vi "linear interp -- residue.vi"(7 "what":enum16{"linear", "quadratic", "nothing"}(ring), 10 "what points in":dbl[](array[numeric])=[-1.4233131928950045, -1.44696698189356, -1.4387793191620561, -1.4336803765711887, -1.4766437914412072, -1.4238891039751602, -1.4266641580299324, -1.4249276723821875, -1.4343882731939412, -1.4156687737284692, -1.4512421695222957, -1.429807437000274, -1.4155556909308238, -1.4387793191620561, -1.4256214336829176, -1.4378261347313517, -1.472241245575028, -1.476513665752772, -1.4669909756005146, -1.430275048869841, -1.4314462860465573, -1.4375881651462725, -1.4885177094699984, -1.3721223035160284, -1.4390179425097644, -1.430626088480954, -1.4084901891013457, -1.4885177094699984, -1.430275048869841, -1.4816176825506562, -1.4117282912536708, -1.420102128492896, -1.414200989082999, -1.4412914275628341, -1.4275931305379441, -1.4362816581303222, -1.4294570582141024, -1.449038245797824, -1.4286406053421603, -1.431211785780653, -1.4307431647673898, -1.430626088480954, -1.4310945831131212, -1.4301580986922384, -1.4330913428691965, -1.5284149439108103, -1.450996736070212, -1.449404790606672, -1.4596705233051261, -1.4422522564545317, -1.4500163869363112, -1.4513649382812484, -1.4485500001231248, -1.4439388390864674, -1.4579218517603743, -1.4631891321044586, -1.465593098958123, -1.4559319537457243, -1.4673729968671088, -1.447210147903218, -1.447696888757646, -1.4348608461262105, -1.447696888757646, -1.4373503258840832, -1.438898614446944, -1.4737899942543355, -1.4484280244217462, -1.4242350175592806, -1.4386600566370986, -1.5039010059634286, -1.4487940543480937, -1.4347426546757862, -1.4293403280744659, -1.4346244953819263, -1.4560560556130935, -1.486382924308125, -1.4525945384285102, -1.5065419471008115, -1.4360445331001872, -1.4326206904450212, -1.4059390968255816, -1.4248121531683389, -1.4270122898977948, -1.4435768767247146, -1.447696888757646, -1.4271283958955197, -1.4268962149320088, -1.4462382997059955, -1.4219341142599085, -1.425968730368281, -1.438540826854084, -1.423773860646395, -1.4007721353222036, -1.4364002692144688, -1.4378261347313517, -1.4333268604898834, -1.4255057298106724, -1.4776862029393325, -1.4273607010531868, -1.4207882178645008, -1.4189610493238327, -1.42969061266012, -1.4112802184959434, -1.4282911662873123, -1.4605475065465392, -1.4270122898977948, -1.394479474658531, -1.4281747490551708, -1.4212462136695654, -1.4236586478902071, -1.407823240700133, -1.4039529905505608, -1.4082677591441644, -1.4256214336829176, -1.41016205494854, -1.4115041970887898, -1.413187728652624, -1.411840381712908, -1.404944908336696, -1.4094925360874166, -1.4263163050022019, -1.4189610493238327, -1.4191890254350537, -1.4124012683747549, -1.4031830621804093, -1.4027437151708582, -1.399462703731531, -1.4038429171798275, -1.4124012683747549, -1.4015377976218495, -1.3966390737476193, -1.4086014468147512, -1.3976144079908948, -1.398265849835895, -1.4081565868712154, -1.3873220797794983, -1.396206293959037, -1.4042833781525756, -1.3759242669503173, -1.3791355228308788, -1.384365529218584, -1.4086014468147512, -1.3885953603844066, -1.402633947829972, -1.3902988957166005, -1.3972890531384425, -1.400007820511902, -1.3731465834292742, -1.376440608090563, -1.4293403280744659, -1.3726341415032672, -1.3798639431222424, -1.3880643730558775, -1.3630108962837708, -1.3713046153819766, -1.392009139548825, -1.3360165434877334, -1.3750993958915096, -1.3514448424333292, -1.3759242669503173, -1.372224622866697, -1.3371477648312038, -1.3381873125587387, -1.3768541234580602, -1.3643152355487773, -1.3590219407376678, -1.3521282327897675, -1.3731465834292742, -1.3689623015592596, -1.3502758121664775, -1.3365817858433202, -1.3120253780614444, -1.3605135088274138, -1.3602147851091797, -1.3516399871150684, -1.3737623129490995, -1.35261702798138, -1.3653212459173176, -1.351835219521999, -1.3320803127786385, -1.372736581527779, -1.410608974959067, -1.3461124400250224, -1.4067139310755428, -1.308830063964396, -1.3486250541829568, -1.3950183684885684, -1.349304018335389, -1.3283644014938703, -1.3056580877318187, -1.3363932899714797, -1.3342314473766201, -1.3269790909671038, -1.3485281458969576, -1.3613111114058765, -1.3408447171553701, -1.330962197210844, -1.324863493628006, -1.3103360330802296, -1.3067128410903444, -1.3183969993651314, -1.3216637513638199, -1.32947584031392, -1.3245883043811366], 11 "temperature points in":dbl[](array[numeric])=[55.393, 55.473, 55.549, 55.623, 55.697, 55.77, 55.847, 55.926, 56.007, 56.087, 56.169, 56.251, 56.332, 56.409, 56.489, 56.565, 56.645, 56.724, 56.8, 56.877, 56.955, 57.034, 57.114, 57.191, 57.269, 57.348, 57.425, 57.505, 57.583, 57.656, 57.736, 57.815, 57.896, 57.974, 58.055, 58.137, 58.217, 58.295, 58.373, 58.45, 58.526, 58.605, 58.679, 58.759, 58.836, 58.913, 58.989, 59.071, 59.148, 59.226, 59.302, 59.381, 59.459, 59.539, 59.616, 59.694, 59.77, 59.846, 59.925, 59.998, 60.076, 60.154, 60.23, 60.308, 60.384, 60.462, 60.54, 60.618, 60.693, 60.77, 60.849, 60.928, 61.004, 61.082, 61.16, 61.239, 61.315, 61.391, 61.468, 61.544, 61.626, 61.703, 61.781, 61.86, 61.93, 62.009, 62.083, 62.162, 62.238, 62.312, 62.389, 62.466, 62.541, 62.618, 62.697, 62.774, 62.854, 63.013, 63.088, 63.165, 63.241, 63.317, 63.394, 63.472, 63.549, 63.628, 63.705, 63.782, 63.861, 63.937, 64.014, 64.089, 64.162, 64.239, 64.316, 64.393, 64.47, 64.547, 64.62, 64.696, 64.817, 64.892, 64.971, 65.046, 65.123, 65.2, 65.275, 65.35, 65.429, 65.507, 65.582, 65.655, 65.733, 65.81, 65.887, 65.965, 66.042, 66.193, 66.27, 66.345, 66.423, 66.5, 66.574, 66.651, 66.728, 66.802, 66.881, 66.956, 67.032, 67.108, 67.187, 67.258, 67.335, 67.411, 67.487, 67.563, 67.639, 67.717, 67.792, 67.869, 67.941, 68.018, 68.097, 68.174, 68.251, 68.349, 68.484, 68.558, 68.632, 68.708, 68.787, 68.864, 69.014, 69.092, 69.169, 69.246, 69.323, 69.397, 69.472, 69.546, 69.621, 69.696, 69.771, 69.845, 69.924, 69.997, 70.071, 70.149, 70.225, 70.301, 70.381, 70.457, 70.533, 70.609, 70.682, 70.76, 70.84, 70.915, 70.993, 71.145, 71.222, 71.3, 71.374, 71.452]) -> (0 "resudue points out":dbl[](array[numeric])=[-1.4233131928950045, -1.44696698189356, -1.4387793191620561, -1.4336803765711887, -1.4766437914412072, -1.4238891039751602, -1.4266641580299324, -1.4249276723821875, -1.4343882731939412, -1.4156687737284692, -1.4512421695222957, -1.429807437000274, -1.4155556909308238, -1.4387793191620561, -1.4256214336829176, -1.4378261347313517, -1.472241245575028, -1.476513665752772, -1.4669909756005146, -1.430275048869841, -1.4314462860465573, -1.4375881651462725, -1.4885177094699984, -1.3721223035160284, -1.4390179425097644, -1.430626088480954, -1.4084901891013457, -1.4885177094699984, -1.430275048869841, -1.4816176825506562, -1.4117282912536708, -1.420102128492896, -1.414200989082999, -1.4412914275628341, -1.4275931305379441, -1.4362816581303222, -1.4294570582141024, -1.449038245797824, -1.4286406053421603, -1.431211785780653, -1.4307431647673898, -1.430626088480954, -1.4310945831131212, -1.4301580986922384, -1.4330913428691965, -1.5284149439108103, -1.450996736070212, -1.449404790606672, -1.4596705233051261, -1.4422522564545317, -1.4500163869363112, -1.4513649382812484, -1.4485500001231248, -1.4439388390864674, -1.4579218517603743, -1.4631891321044586, -1.465593098958123, -1.4559319537457243, -1.4673729968671088, -1.447210147903218, -1.447696888757646, -1.4348608461262105, -1.447696888757646, -1.4373503258840832, -1.438898614446944, -1.4737899942543355, -1.4484280244217462, -1.4242350175592806, -1.4386600566370986, -1.5039010059634286, -1.4487940543480937, -1.4347426546757862, -1.4293403280744659, -1.4346244953819263, -1.4560560556130935, -1.486382924308125, -1.4525945384285102, -1.5065419471008115, -1.4360445331001872, -1.4326206904450212, -1.4059390968255816, -1.4248121531683389, -1.4270122898977948, -1.4435768767247146, -1.447696888757646, -1.4271283958955197, -1.4268962149320088, -1.4462382997059955, -1.4219341142599085, -1.425968730368281, -1.438540826854084, -1.423773860646395, -1.4007721353222036, -1.4364002692144688, -1.4378261347313517, -1.4333268604898834, -1.4255057298106724, -1.4776862029393325, -1.4273607010531868, -1.4207882178645008, -1.4189610493238327, -1.42969061266012, -1.4112802184959434, -1.4282911662873123, -1.4605475065465392, -1.4270122898977948, -1.394479474658531, -1.4281747490551708, -1.4212462136695654, -1.4236586478902071, -1.407823240700133, -1.4039529905505608, -1.4082677591441644, -1.4256214336829176, -1.41016205494854, -1.4115041970887898, -1.413187728652624, -1.411840381712908, -1.404944908336696, -1.4094925360874166, -1.4263163050022019, -1.4189610493238327, -1.4191890254350537, -1.4124012683747549, -1.4031830621804093, -1.4027437151708582, -1.399462703731531, -1.4038429171798275, -1.4124012683747549, -1.4015377976218495, -1.3966390737476193, -1.4086014468147512, -1.3976144079908948, -1.398265849835895, -1.4081565868712154, -1.3873220797794983, -1.396206293959037, -1.4042833781525756, -1.3759242669503173, -1.3791355228308788, -1.384365529218584, -1.4086014468147512, -1.3885953603844066, -1.402633947829972, -1.3902988957166005, -1.3972890531384425, -1.400007820511902, -1.3731465834292742, -1.376440608090563, -1.4293403280744659, -1.3726341415032672, -1.3798639431222424, -1.3880643730558775, -1.3630108962837708, -1.3713046153819766, -1.392009139548825, -1.3360165434877334, -1.3750993958915096, -1.3514448424333292, -1.3759242669503173, -1.372224622866697, -1.3371477648312038, -1.3381873125587387, -1.3768541234580602, -1.3643152355487773, -1.3590219407376678, -1.3521282327897675, -1.3731465834292742, -1.3689623015592596, -1.3502758121664775, -1.3365817858433202, -1.3120253780614444, -1.3605135088274138, -1.3602147851091797, -1.3516399871150684, -1.3737623129490995, -1.35261702798138, -1.3653212459173176, -1.351835219521999, -1.3320803127786385, -1.372736581527779, -1.410608974959067, -1.3461124400250224, -1.4067139310755428, -1.308830063964396, -1.3486250541829568, -1.3950183684885684, -1.349304018335389, -1.3283644014938703, -1.3056580877318187, -1.3363932899714797, -1.3342314473766201, -1.3269790909671038, -1.3485281458969576, -1.3613111114058765, -1.3408447171553701, -1.330962197210844, -1.324863493628006, -1.3103360330802296, -1.3067128410903444, -1.3183969993651314, -1.3216637513638199, -1.32947584031392, -1.3245883043811366], 2 "what points out":dbl[](array[numeric])=[-1.4233131928950045, -1.44696698189356, -1.4387793191620561, -1.4336803765711887, -1.4766437914412072, -1.4238891039751602, -1.4266641580299324, -1.4249276723821875, -1.4343882731939412, -1.4156687737284692, -1.4512421695222957, -1.429807437000274, -1.4155556909308238, -1.4387793191620561, -1.4256214336829176, -1.4378261347313517, -1.472241245575028, -1.476513665752772, -1.4669909756005146, -1.430275048869841, -1.4314462860465573, -1.4375881651462725, -1.4885177094699984, -1.3721223035160284, -1.4390179425097644, -1.430626088480954, -1.4084901891013457, -1.4885177094699984, -1.430275048869841, -1.4816176825506562, -1.4117282912536708, -1.420102128492896, -1.414200989082999, -1.4412914275628341, -1.4275931305379441, -1.4362816581303222, -1.4294570582141024, -1.449038245797824, -1.4286406053421603, -1.431211785780653, -1.4307431647673898, -1.430626088480954, -1.4310945831131212, -1.4301580986922384, -1.4330913428691965, -1.5284149439108103, -1.450996736070212, -1.449404790606672, -1.4596705233051261, -1.4422522564545317, -1.4500163869363112, -1.4513649382812484, -1.4485500001231248, -1.4439388390864674, -1.4579218517603743, -1.4631891321044586, -1.465593098958123, -1.4559319537457243, -1.4673729968671088, -1.447210147903218, -1.447696888757646, -1.4348608461262105, -1.447696888757646, -1.4373503258840832, -1.438898614446944, -1.4737899942543355, -1.4484280244217462, -1.4242350175592806, -1.4386600566370986, -1.5039010059634286, -1.4487940543480937, -1.4347426546757862, -1.4293403280744659, -1.4346244953819263, -1.4560560556130935, -1.486382924308125, -1.4525945384285102, -1.5065419471008115, -1.4360445331001872, -1.4326206904450212, -1.4059390968255816, -1.4248121531683389, -1.4270122898977948, -1.4435768767247146, -1.447696888757646, -1.4271283958955197, -1.4268962149320088, -1.4462382997059955, -1.4219341142599085, -1.425968730368281, -1.438540826854084, -1.423773860646395, -1.4007721353222036, -1.4364002692144688, -1.4378261347313517, -1.4333268604898834, -1.4255057298106724, -1.4776862029393325, -1.4273607010531868, -1.4207882178645008, -1.4189610493238327, -1.42969061266012, -1.4112802184959434, -1.4282911662873123, -1.4605475065465392, -1.4270122898977948, -1.394479474658531, -1.4281747490551708, -1.4212462136695654, -1.4236586478902071, -1.407823240700133, -1.4039529905505608, -1.4082677591441644, -1.4256214336829176, -1.41016205494854, -1.4115041970887898, -1.413187728652624, -1.411840381712908, -1.404944908336696, -1.4094925360874166, -1.4263163050022019, -1.4189610493238327, -1.4191890254350537, -1.4124012683747549, -1.4031830621804093, -1.4027437151708582, -1.399462703731531, -1.4038429171798275, -1.4124012683747549, -1.4015377976218495, -1.3966390737476193, -1.4086014468147512, -1.3976144079908948, -1.398265849835895, -1.4081565868712154, -1.3873220797794983, -1.396206293959037, -1.4042833781525756, -1.3759242669503173, -1.3791355228308788, -1.384365529218584, -1.4086014468147512, -1.3885953603844066, -1.402633947829972, -1.3902988957166005, -1.3972890531384425, -1.400007820511902, -1.3731465834292742, -1.376440608090563, -1.4293403280744659, -1.3726341415032672, -1.3798639431222424, -1.3880643730558775, -1.3630108962837708, -1.3713046153819766, -1.392009139548825, -1.3360165434877334, -1.3750993958915096, -1.3514448424333292, -1.3759242669503173, -1.372224622866697, -1.3371477648312038, -1.3381873125587387, -1.3768541234580602, -1.3643152355487773, -1.3590219407376678, -1.3521282327897675, -1.3731465834292742, -1.3689623015592596, -1.3502758121664775, -1.3365817858433202, -1.3120253780614444, -1.3605135088274138, -1.3602147851091797, -1.3516399871150684, -1.3737623129490995, -1.35261702798138, -1.3653212459173176, -1.351835219521999, -1.3320803127786385, -1.372736581527779, -1.410608974959067, -1.3461124400250224, -1.4067139310755428, -1.308830063964396, -1.3486250541829568, -1.3950183684885684, -1.349304018335389, -1.3283644014938703, -1.3056580877318187, -1.3363932899714797, -1.3342314473766201, -1.3269790909671038, -1.3485281458969576, -1.3613111114058765, -1.3408447171553701, -1.330962197210844, -1.324863493628006, -1.3103360330802296, -1.3067128410903444, -1.3183969993651314, -1.3216637513638199, -1.32947584031392, -1.3245883043811366], 3 "temperature points OUT":dbl[](array[numeric])=[55.393, 55.473, 55.549, 55.623, 55.697, 55.77, 55.847, 55.926, 56.007, 56.087, 56.169, 56.251, 56.332, 56.409, 56.489, 56.565, 56.645, 56.724, 56.8, 56.877, 56.955, 57.034, 57.114, 57.191, 57.269, 57.348, 57.425, 57.505, 57.583, 57.656, 57.736, 57.815, 57.896, 57.974, 58.055, 58.137, 58.217, 58.295, 58.373, 58.45, 58.526, 58.605, 58.679, 58.759, 58.836, 58.913, 58.989, 59.071, 59.148, 59.226, 59.302, 59.381, 59.459, 59.539, 59.616, 59.694, 59.77, 59.846, 59.925, 59.998, 60.076, 60.154, 60.23, 60.308, 60.384, 60.462, 60.54, 60.618, 60.693, 60.77, 60.849, 60.928, 61.004, 61.082, 61.16, 61.239, 61.315, 61.391, 61.468, 61.544, 61.626, 61.703, 61.781, 61.86, 61.93, 62.009, 62.083, 62.162, 62.238, 62.312, 62.389, 62.466, 62.541, 62.618, 62.697, 62.774, 62.854, 63.013, 63.088, 63.165, 63.241, 63.317, 63.394, 63.472, 63.549, 63.628, 63.705, 63.782, 63.861, 63.937, 64.014, 64.089, 64.162, 64.239, 64.316, 64.393, 64.47, 64.547, 64.62, 64.696, 64.817, 64.892, 64.971, 65.046, 65.123, 65.2, 65.275, 65.35, 65.429, 65.507, 65.582, 65.655, 65.733, 65.81, 65.887, 65.965, 66.042, 66.193, 66.27, 66.345, 66.423, 66.5, 66.574, 66.651, 66.728, 66.802, 66.881, 66.956, 67.032, 67.108, 67.187, 67.258, 67.335, 67.411, 67.487, 67.563, 67.639, 67.717, 67.792, 67.869, 67.941, 68.018, 68.097, 68.174, 68.251, 68.349, 68.484, 68.558, 68.632, 68.708, 68.787, 68.864, 69.014, 69.092, 69.169, 69.246, 69.323, 69.397, 69.472, 69.546, 69.621, 69.696, 69.771, 69.845, 69.924, 69.997, 70.071, 70.149, 70.225, 70.301, 70.381, 70.457, 70.533, 70.609, 70.682, 70.76, 70.84, 70.915, 70.993, 71.145, 71.222, 71.3, 71.374, 71.452])   [LabVIEW 2014]
uses:
  <vilib>/Analysis/baseanly.llb/A x B.vi
  <vilib>/Analysis/baseanly.llb/Real A x B.vi
  Q -- check range -- i -- real.vi
  Q -- check range -- i -- integer.vi
  Q - not nan -- real.vi
  Q - not nan -- integer.vi
  <vilib>/Analysis/Matrix/Numeric/Conversions/Array To Matrix.vi
  <vilib>/Analysis/Matrix/Numeric/Conversions/Array To Matrix - RA2.vi
  <vilib>/Analysis/baseanly.llb/Inverse Matrix.vi
  <vilib>/Analysis/baseanly.llb/Real Inverse Matrix.vi
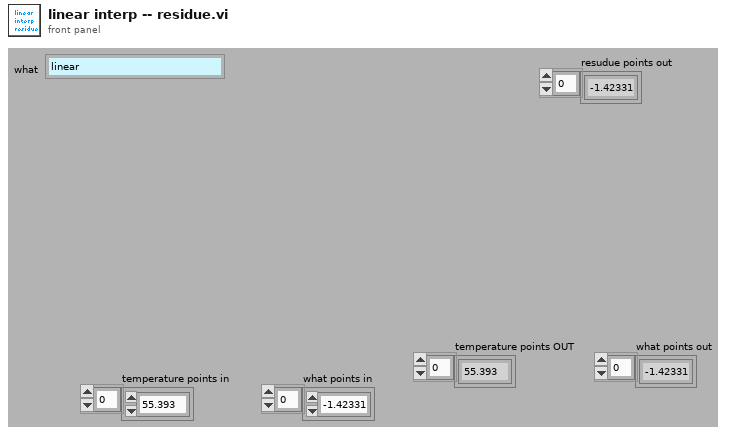
[diagram p1: front panel]
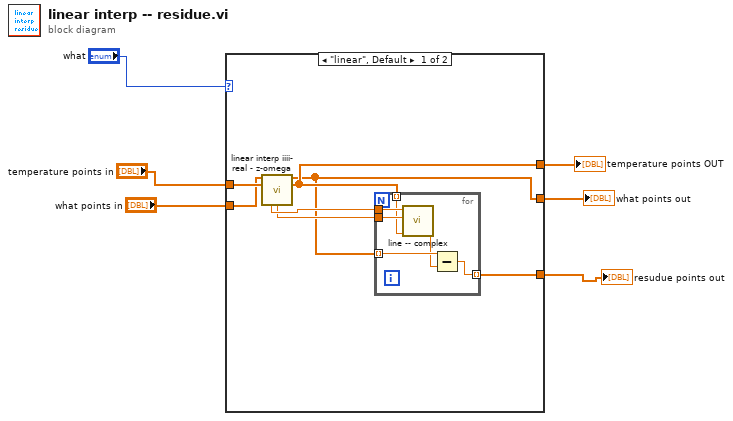
[diagram p0: block diagram]
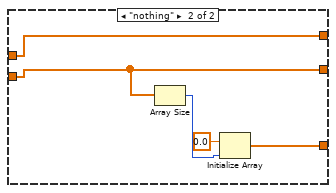
[diagram p2: hidden frame]
diagram:
  n1 = case shown="\"linear\", Default" "what" {
    tunnel: "temperature points in" -> [w13 w24]
    tunnel: "what points in" -> [w12 w22]
    tunnel: [w9 w24] -> w3
    tunnel: [w8 w22] -> w2
    tunnel: [w7 w20] -> w1
    frame "linear", Default {
      n2 = call "linear interp iiii- real - z-omega.vi"("z"=w12, "omega"=w13) -> ("z out"=w8:dbl[], "omega out"=w9:dbl[], "intercept"=w11:dbl, "slope"=w10:dbl)  [unwired: 4 in, 6 out]
      n3 = for {
        tunnel: w11 -> [w19]
        tunnel: w10 -> [w18]
        tunnel: w9 -> [w17] mode=indexing
        tunnel: w8 -> [w16] mode=indexing
        tunnel: [w14] -> w7 mode=indexing
        n4 = call "line -- complex.vi"("n"=w17, "slope"=w18, "intercept"=w19) -> ("value"=w15:cdb)  [unwired: 7 in, 1 out]
        n5 = Subtract(x=w16, y=w15) -> (x-y=w14:cdb)
      }
    }
    frame "nothing" {
      n6 = Array Size(array=w22) -> (size(s)=w21:i32)
      n7 = Initialize Array(0.0 ("element"), w21) -> (w20:dbl[])
    }
  }
  "temperature points OUT" <- w3
  "what points out" <- w2
  "resudue points out" <- w1
